vi "UTIL_dynamic Error logger start v1_0_0.vi"(8 "error in (no error)":errorcluster, 10 "Error File Path":path=path "C:/Error Log.txt", 11 "Error.vi Path":path) -> (0 "error out":errorcluster, 3 "Error Ref out":refnum<vi>)   [LabVIEW 2009]
doc: "Util_dynamic Error logger start.vi\n\nThis vi is used to dynamically start the Error Q.vi. use it to cleanly launch error logger. \n\nCreated 2006 by:\n\nJ. Daren Suntych\nNational Analytics\n970-397-0764"
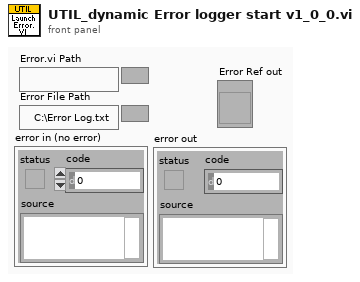
[diagram p1: front panel]
types:
  T1 = enum32{"Invalid", "Standard", "Closed", "Hidden", "Minimized", "Maximized"}
  T2 = enum32{"Bad", "Idle", "Run top level", "Running"}
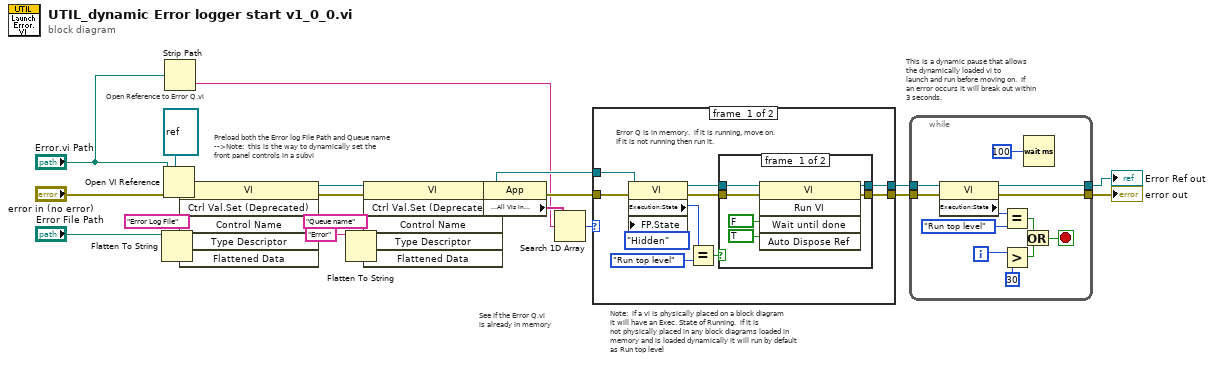
[diagram p0: block diagram]
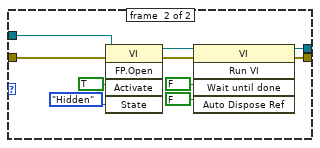
[diagram p3: hidden frame]
diagram:
  # "This is a dynamic pause that allows\nthe dynamically loaded vi to \nlaunch and run before moving on.  If \nan error occurs it will break out within\n3 seconds."
  # "Note:  if a vi is physically placed on a block diagram\nit will have an Exec. State of Running.  if it is\nnot physically placed in any block diagrams loaded in\nmemory and is loaded dynamically it will run by default\nas Run top level"
  # "Preload both the Error log File Path and Queue name\n-->Note:  this is the way to dynamically set the \nfront panel controls in a subvi"
  # "Open Reference to Error Q.vi"
  # "See if the Error Q.vi\nis already in memory"
  n1 = Flatten To String(anything="Error File Path") -> (data string=w21:string, type string=w22:i16[])  [unwired: 1 in, 3 out]
  n2 = Open VI Reference(type specifier VI Refnum (for type only)=refnum<vi> refnum, vi path="Error.vi Path", error in (no error)="error in (no error)") -> (vi reference=w25:refnum<vi>, error out=w24:errorcluster)  [unwired: 3 out]
  n3 = Strip Path(path="Error.vi Path") -> (name=w1:string)  [unwired: 1 out]
  n4 = invoke class="VI" method="Ctrl Val.Set (Deprecated)"(reference=w25, error in=w24, "Control Name"="Error Log File", "Type Descriptor"=w22, "Flattened Data"=w21) -> (reference out=w4:refnum<vi>, error out=w7:errorcluster)  [unwired: 1 in, 4 out]
  n5 = Flatten To String(anything="Error" ("Control Name")) -> (data string=w10:string, type string=w9:i16[])  [unwired: 1 in, 3 out]
  n6 = invoke class="VI" method="Ctrl Val.Set (Deprecated)"(reference=w4, error in=w7, "Control Name"="Queue name", "Type Descriptor"=w9, "Flattened Data"=w10) -> (reference out=w5:refnum<vi>, error out=w6:errorcluster)  [unwired: 1 in, 4 out]
  n7 = property class="App"(error in=w6) -> (error out=w11:errorcluster, "Application:All VIs In Memory"=w18:string[])  [unwired: 1 in, 1 out]
  n8 = Search 1D Array(1D array=w18, element=w1) -> (index of element=w17:i32)  [unwired: 1 out]
  n9 = case shown="-1" w17 {
    tunnel: w11 -> [w33 w53]
    tunnel: [w35 w45] -> w14
    tunnel: [w34 w47] -> w13
    tunnel: w5 -> [w27 w44]
    frame #0 {
      # "Error Q is in memory.  if it is running, move on.\nIf it is not running then run it."
      n10 = property class="VI"(reference=w27, error in=w33, "FP.State"=T1."Hidden" ("Front Panel Window:State")) -> (reference out=w31:refnum<vi>, error out=w32:errorcluster, "Execution:State"=w30:T2)
      n11 = Equal?(x=w30, y=T2."Run top level") -> (x = y?=w28:bool)
      n12 = case shown="False" w28 {
        tunnel: [w40 w42] -> w35
        tunnel: [w39 w43] -> w34
        tunnel: w32 -> [w38 w42]
        tunnel: w31 -> [w37 w43]
        frame #0 {
          n13 = invoke class="VI" method="Run VI"(reference=w37, error in=w38, "Wait until done"=FALSE, "Auto Dispose Ref"=TRUE ("Wait until done")) -> (reference out=w39:refnum<vi>, error out=w40:errorcluster)  [unwired: 1 in, 3 out]
        }
        frame #1 {
        }
      }
    }
    frame #1 {
      n14 = invoke class="VI" method="FP.Open"(reference=w44, error in=w53, "Activate"=TRUE, "State"=T1."Hidden") -> (reference out=w48:refnum<vi>, error out=w46:errorcluster)  [unwired: 1 in, 3 out]
      n15 = invoke class="VI" method="Run VI"(reference=w48, error in=w46, "Wait until done"=FALSE, "Auto Dispose Ref"=FALSE ("Wait until done")) -> (reference out=w47:refnum<vi>, error out=w45:errorcluster)  [unwired: 1 in, 3 out]
    }
  }
  n16 = while {
    tunnel: w13 -> [w65]
    tunnel: w14 -> [w64]
    tunnel: [w56] -> w16
    tunnel: [w54] -> w15
    i -> [w61]
    stop <- w57 stop-if-true
    n17 = property class="VI"(reference=w65, error in=w64) -> (reference out=w54:refnum<vi>, error out=w56:errorcluster, "Execution:State"=w63:T2)
    n18 = Equal?(x=w63, y=T2."Run top level" ("Execution:State")) -> (x = y?=w59:bool)
    n19 = Greater?(x=w61, y=30) -> (0:w58:bool)
    n20 = Or(x=w59, y=w58) -> (x .or. y?=w57:bool)
    n21 = Wait (ms)(milliseconds to wait=u32 100) -> ()  [unwired: 1 out]
  }
  "error out" <- w16
  "Error Ref out" <- w15
